vi "sort_arrays.vi"(2 "index":i32[](array[numeric]), 3 "string":string[](array[string])) -> (0 "index 2":i32[](array[numeric]), 1 "string 2":string[](array[string]))   [LabVIEW 2014]
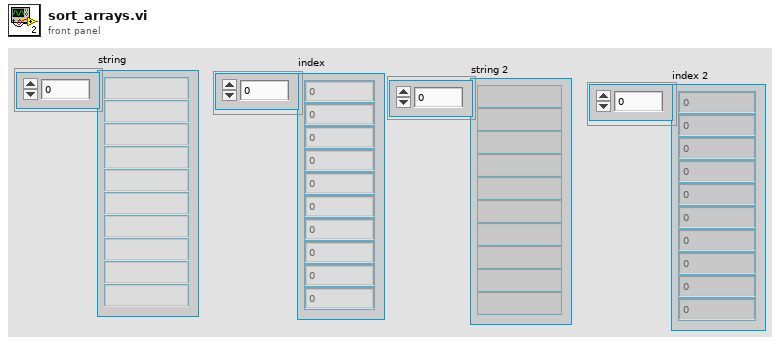
[diagram p1: front panel]
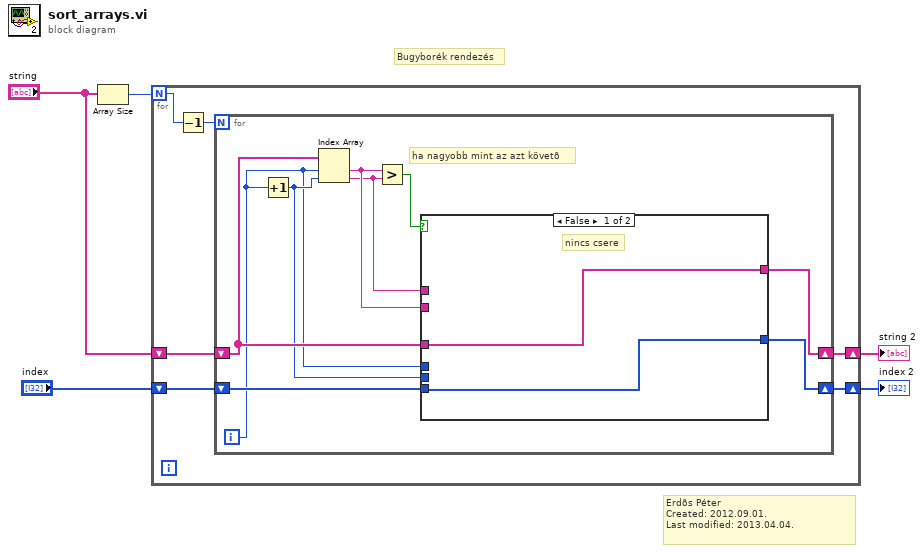
[diagram p0: block diagram]
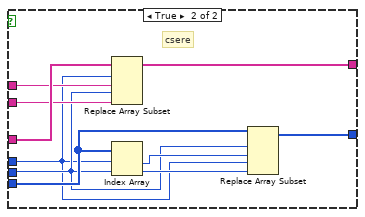
[diagram p2: hidden frame]
diagram:
  # "Erdõs Péter\nCreated: 2012.09.01.\nLast modified: 2013.04.04."
  # "Bugyborék rendezés"
  n1 = Array Size(array="string") -> (size(s)=w5:i32)
  n2 = for {
    N: w5 -> [w10]
    shift-right: [w8] -> w3
    shift-left: "string" -> [w9]
    shift-right: [w6] -> w1
    shift-left: "index" -> [w7]
    n3 = Decrement(x=w10) -> (x-1=w11:i32)
    n4 = for {
      N: w11 -> [_]
      shift-right: [w18] -> w8
      shift-left: w9 -> [w19]
      shift-right: [w16] -> w6
      shift-left: w7 -> [w17]
      i -> [w13]
      # "ha nagyobb mint az azt követõ"
      n5 = Increment(x=w13) -> (x+1=w15:i32)
      n6 = Index Array(array=w19, index #1=w13, index #2=w15) -> (element #1=w14:string, element #2=w12:string)
      n7 = Greater?(x=w14, y=w12) -> (0:w20:bool)
      n8 = case shown="False" w20 {
        tunnel: w19 -> [w22 w32]
        tunnel: [w22 w31] -> w18
        tunnel: w17 -> [w21 w29]
        tunnel: [w21 w30] -> w16
        tunnel: w13 -> [_ w23]
        tunnel: w15 -> [_ w24]
        tunnel: w12 -> [_ w28]
        tunnel: w14 -> [_ w27]
        frame False {
          # "nincs csere"
        }
        frame True {
          # "csere"
          n9 = Replace Array Subset(array=w32, new element #1=w28, index #1=w23, new element #2=w27, index #2=w24) -> (w31:string[])
          n10 = Index Array(array=w29, index #1=w23, index #2=w24) -> (element #1=w25:i32, element #2=w26:i32)
          n11 = Replace Array Subset(array=w29, new element #1=w25, index #1=w24, new element #2=w26, index #2=w23) -> (w30:i32[])
        }
      }
    }
  }
  "string 2" <- w3
  "index 2" <- w1
